vi "StringDecoder.vi"(10 "Auto Config File":path=path "C:/Users/Matthew/Desktop/Auto Config Testing/autoexample.txt") -> ()   [LabVIEW 2014]
uses:
  Shared/MethodCluster.ctl
panel:
  out "Method Cluster":T1
  out "Should Stop?":bool
  out "Extra Lines Removed":string[](array[string])
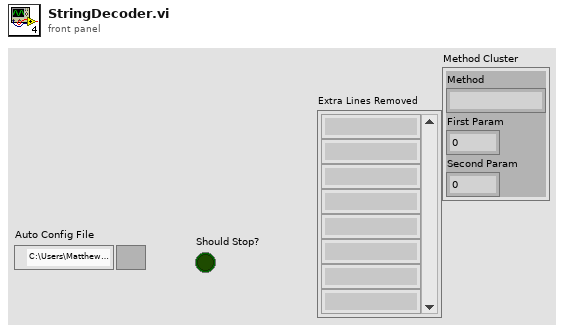
[diagram p1: front panel]
types:
  T1 = typedef "MethodCluster.ctl" = cluster{"Method":string, "First Param":dbl, "Second Param":dbl}
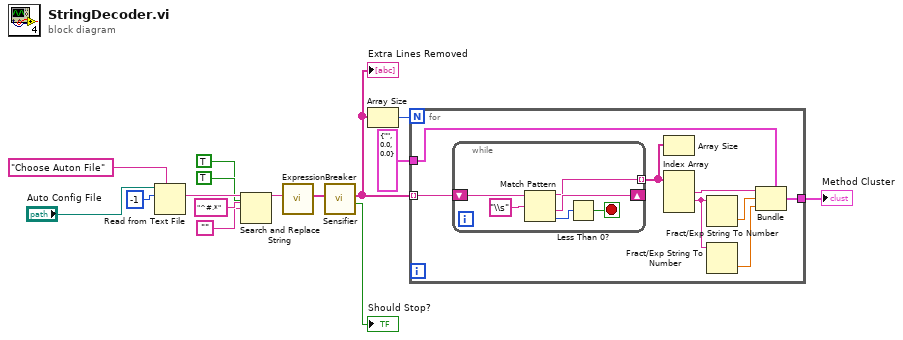
[diagram p0: block diagram]
diagram:
  n1 = Read from Text File(prompt (Open existing file)="Choose Auton File", file (use dialog)="Auto Config File", count=-1) -> (text=w13:string)  [unwired: 1 in, 3 out]
  n2 = Search and Replace String(replace all?=TRUE ("replace all? (F)"), multiline?=TRUE ("multiline? (F)"), input string=w13, search string="^#.*" ("regular expression"), replace string="") -> (result string=w6:string)  [unwired: 3 in, 3 out]
  n3 = call "ExpressionBreaker.vi"("result string"=w6) -> ("Broken Strings"=w5:string[])  [unwired: 10 in]
  n4 = call "Sensifier.vi"("Array"=w5) -> ("Has Errors?"=→"Should Stop?":bool, "Sensed"=w3:string[])  [unwired: 9 in]
  "Extra Lines Removed" <- w3
  n5 = Array Size(array=w3) -> (size(s)=w4:i32)
  n6 = for {
    N: w4 -> [_]
    tunnel: w3 -> [w23] mode=indexing
    tunnel: T1 {"Method"="", "First Param"=0.0, "Second Param"=0.0} ("Method Cluster") -> [w21]
    tunnel: [w20] -> w2
    n7 = while {
      shift-right: [w27] -> _
      shift-left: w23 -> [w28]
      tunnel: [w26] -> w22 mode=indexing
      stop <- w25 stop-if-true
      n8 = Match Pattern(string=w28, regular expression="\\s") -> (before substring=w26:string, after substring=w27:string, offset past match=w24:i32)  [unwired: 1 in, 1 out]
      n9 = Less Than 0?(x=w24) -> (x < 0?=w25:bool)
    }
    n10 = Array Size(array=w22) -> ()  [unwired: 1 out]
    n11 = Index Array(array=w22) -> (element #1=w19:string, element #2=w17:string)  [unwired: 3 in, 1 out]
    n12 = Fract/Exp String To Number(string=w17) -> (number=w18:dbl)  [unwired: 3 in, 1 out]
    n13 = Fract/Exp String To Number(string=w17) -> (number=w16:dbl)  [unwired: 3 in, 1 out]
    n14 = Bundle(cluster=w21, "Method"=w19, "First Param"=w18, "Second Param"=w16) -> (w20:T1)
  }
  "Method Cluster" <- w2
